vi "Get Individual Values of Voltage or Current.vi"(6 "output function":T1=1007 caption="Output Function" items=["DC Voltage"=1006, "DC Current"=1007, "Pulse Voltage"=1049, "Pulse Current"=1050], 8 "error in (no error)":errorcluster, 10 "Values In":dbl[](array[numeric]), 11 "Ganged Session In":T2) -> (0 "error out":errorcluster, 2 "Values Out":dbl[](array[numeric]), 3 "Ganged Session Out":T2)   [LabVIEW 2021]
uses:
  ctl/NIDCPower_channel_ganging - ctl - ganged session.ctl
  ctl/NIDCPower_channel_ganging - ctl - ganged config.ctl
  ctl/NIDCPower_channel_ganging - ctl - channel mode.ctl
  <instrlib>/niDCPower/nidcpower.llb/niDCPower Output Function.ctl
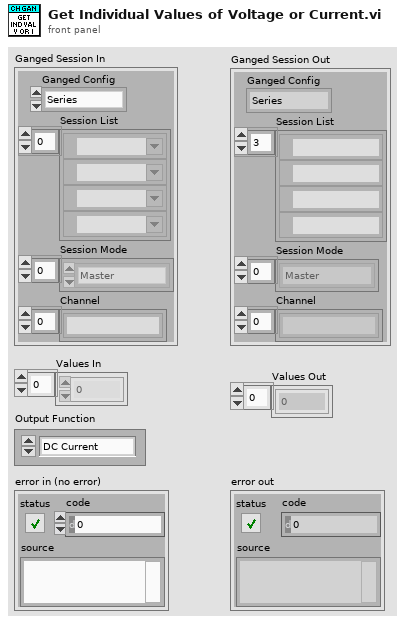
[diagram p1: front panel]
types:
  T1 = typedef "niDCPower Output Function.ctl" = i32
  T2 = typedef "NIDCPower_channel_ganging - ctl - ganged session.ctl" = cluster{"Ganged Config":T3, "Session List":refnum<k15>[], "Session Mode":T4[], "Channel":string[]}
  T3 = typedef "NIDCPower_channel_ganging - ctl - ganged config.ctl" = enum32{"Series", "Parallel", "Manual"}
  T4 = typedef "NIDCPower_channel_ganging - ctl - channel mode.ctl" = enum32{"Master", "Slave", "Slave - Inverted"}
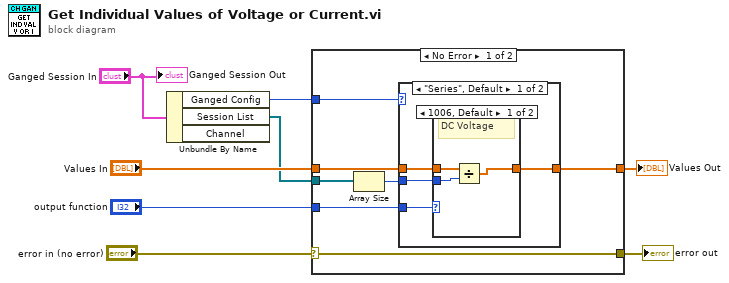
[diagram p0: block diagram]
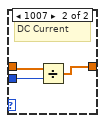
[diagram p4: hidden frame]
diagram:
  n1 = Unbundle By Name("Ganged Session In") -> ("Ganged Config"=w7:T3, "Session List"=w4:refnum<k15>[])  [unwired: 1 out]
  n2 = case shown="No Error" "error in (no error)" {
    selector: "error in (no error)" -> [w10 w32]
    tunnel: w7 -> [w15 _]
    tunnel: "output function" -> [w14 _]
    tunnel: "Values In" -> [w13 _]
    tunnel: w4 -> [w12 _]
    tunnel: [w10 w32] -> w2
    tunnel: [w9 _] -> w1
    frame No Error {
      n3 = Array Size(array=w12) -> (size(s)=w11:i32)
      n4 = case shown="\"Series\", Default" w15 {
        tunnel: w13 -> [w19 w27]
        tunnel: w14 -> [w16 w26]
        tunnel: [w18 w25] -> w9
        tunnel: w11 -> [w17 w24]
        frame "Series", Default {
          n5 = case shown="1006, Default" w16 {
            tunnel: w19 -> [w22 w23]
            tunnel: [w21 w23] -> w18
            tunnel: w17 -> [w20 _]
            frame 1006, Default {
              # "DC Voltage"
              n6 = Divide(x=w22, y=w20) -> (x/y=w21:dbl[])
            }
            frame 1007 {
              # "DC Current"
            }
          }
        }
        frame "Parallel" {
          n7 = case shown="1006, Default" w26 {
            tunnel: w27 -> [w28 w31]
            tunnel: [w28 w29] -> w25
            tunnel: w24 -> [_ w30]
            frame 1006, Default {
              # "DC Voltage"
            }
            frame 1007 {
              # "DC Current"
              n8 = Divide(x=w31, y=w30) -> (x/y=w29:dbl[])
            }
          }
        }
      }
    }
    frame Error {
    }
  }
  "error out" <- w2
  "Values Out" <- w1
  "Ganged Session Out" <- "Ganged Session In"
